vi "TLMB_Get_Latest_Build_From_Artifactory.vi"(7 "Repository":string="CIBuild_TLMB", 11 "Error In":errorcluster) -> (4 "Output Path":path, 8 "Build":string, 15 "Error Out 2":errorcluster)   [LabVIEW 2016, in "TLMB.lvlib"]
uses:
  Projects/TLMB.lvlib
  <vilib>/regexp/Match Regular Expression.xnode
  <vilib>/httpClient/LabVIEWHTTPClient.lvlib
  <vilib>/zip/NI_Unzip.lvlib
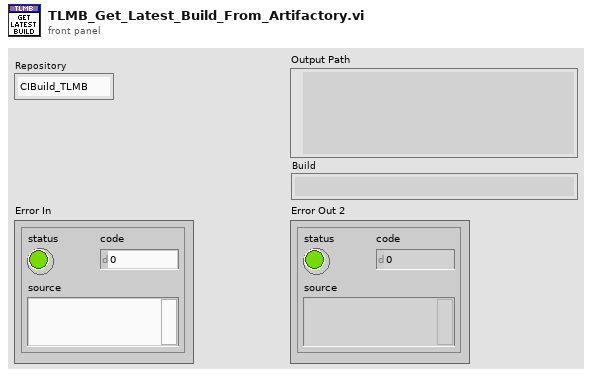
[diagram p1: front panel]
types:
  T1 = typedef "LabVIEWHTTPClient.lvlib/ClientHandle.ctl" = refnum<k1>
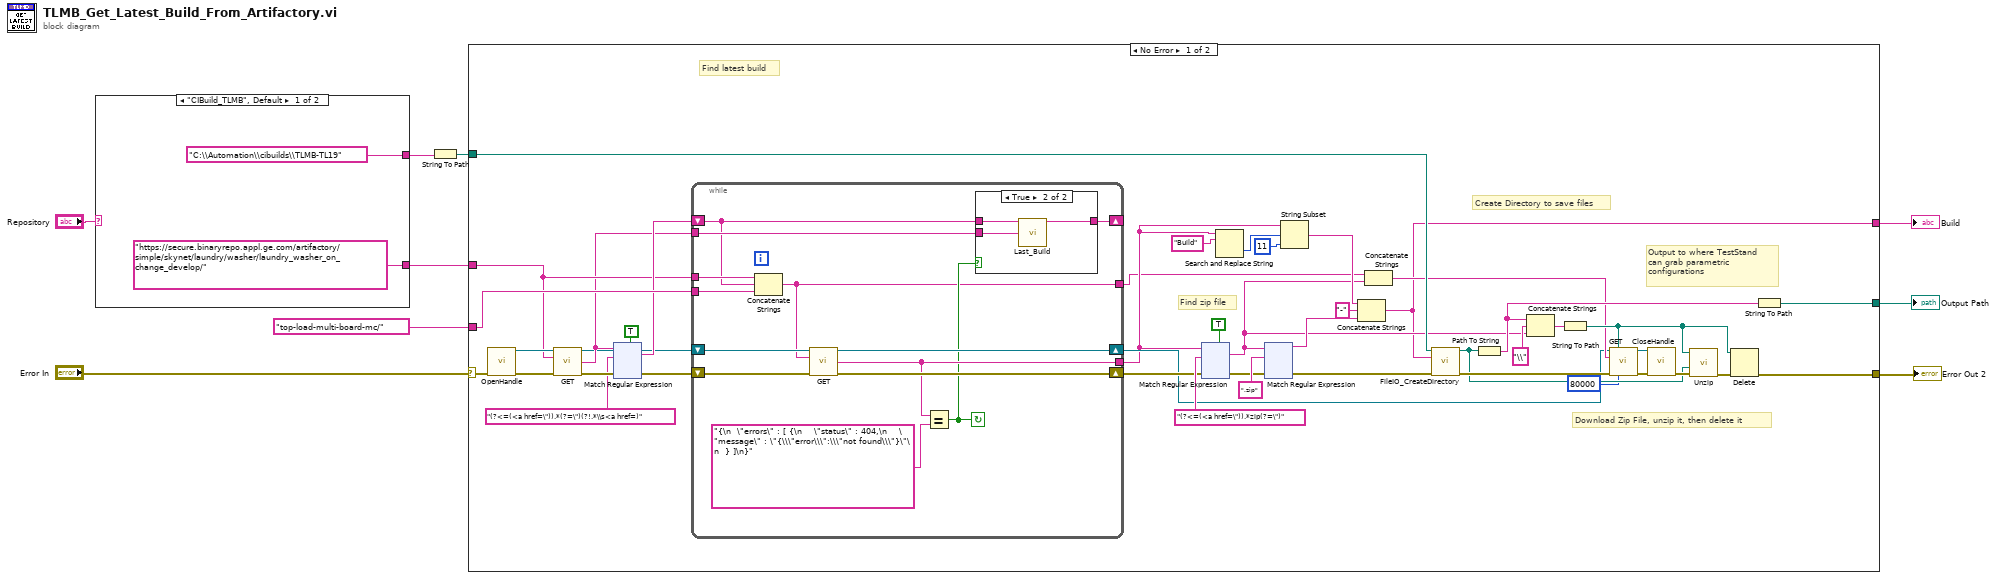
[diagram p0: block diagram]
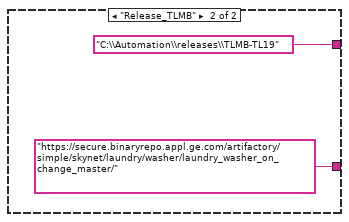
[diagram p2: hidden frame]
diagram:
  n1 = case shown="\"CIBuild_TLMB\", Default" "Repository" {
    tunnel: ["C:\\Automation\\cibuilds\\TLMB-TL19" "C:\\Automation\\releases\\TLMB-TL19"] -> w6
    tunnel: ["https://secure.binaryrepo.appl.ge.com/artifactory/simple/skynet/laundry/washer/laundry_washer_on_change_develop/" ("regular expression") "https://secure.binaryrepo.appl.ge.com/artifactory/simple/skynet/laundry/washer/laundry_washer_on_change_master/" ("regular expression")] -> w3
    frame "CIBuild_TLMB", Default {
    }
    frame "Release_TLMB" {
    }
  }
  n2 = String To Path(string=w6) -> (path=w5:path)
  n3 = case shown="No Error" "Error In" {
    selector: "Error In" -> [w55 w417]
    tunnel: [w40 w417] -> w7
    tunnel: [w35 _] -> w8
    tunnel: w5 -> [w36 _]
    tunnel: w3 -> [w21 _]
    tunnel: "top-load-multi-board-mc/" -> [w23 _]
    tunnel: [w24 _] -> w1
    frame No Error {
      # "Create Directory to save files"
      # "Output to where TestStand\ncan grab parametric\nconfigurations"
      # "Find zip file"
      # "Find latest build"
      # "Download Zip File, unzip it, then delete it"
      n4 = call <vilib>:"OpenHandle.vi"("error in (no error)"=w55) -> ("client handle out"=w56:T1, "error out"=w57:errorcluster)  [unwired: 13 in]
      n5 = call <vilib>:"GET.vi"("client handle"=w56, "url"=w21, "error in (no error)"=w57) -> ("client handle out"=w18:T1, "body"=w20:string, "error out"=w54:errorcluster)  [unwired: 9 in, 1 out]
      n6 = xnode "Match Regular Expression"("input string"=w20, "regular expression"="(?<=(<a href=\")).*(?=\")(?!.*\\s<a href=)", "error in"=w54, "multiline? (F)"=TRUE) -> ("whole match"=w22:string, "error out"=w19:errorcluster)  [unwired: 2 in, 3 out]
      n7 = while {
        shift-right: [w70] -> w17
        shift-left: w19 -> [w68]
        shift-right: [w69] -> w16
        shift-left: w18 -> [w67]
        tunnel: [w65] -> w15
        tunnel: w20 -> [w63]
        shift-right: [w62] -> _
        shift-left: w22 -> [w60]
        tunnel: w21 -> [w61]
        tunnel: [w59] -> w14
        tunnel: w23 -> [w58]
        stop <- w64 continue-if-true
        n8 = Concatenate Strings(w61, w60, w58) -> (w59:string)
        n9 = call <vilib>:"GET.vi"("client handle"=w67, "url"=w59, "error in (no error)"=w68) -> ("client handle out"=w69:T1, "body"=w65:string, "error out"=w70:errorcluster)  [unwired: 9 in, 1 out]
        n10 = Equal?(x=w65, y="{\n  \"errors\" : [ {\n    \"status\" : 404,\n    \"message\" : \"{\\\"error\\\":\\\"not found\\\"}\"\n  } ]\n}") -> (x = y?=w64:bool)
        n11 = case shown="True" w64 {
          tunnel: w63 -> [_ w74]
          tunnel: w60 -> [w71 w73]
          tunnel: [w71 w72] -> w62
          frame False {
          }
          frame True {
            n12 = call "Last_Build.vi"("Current Build"=w73, "Webpage Source"=w74) -> ("Next Build"=w72:string)  [unwired: 13 in]
          }
        }
      }
      n13 = xnode "Match Regular Expression"("input string"=w15, "regular expression"="(?<=(<a href=\")).*zip(?=\")", "error in"=w17, "multiline? (F)"=TRUE) -> ("whole match"=w26:string, "error out"=w44:errorcluster)  [unwired: 2 in, 3 out]
      n14 = Search and Replace String(input string=w15, search string="Build") -> (offset past replacement=w30:i32)  [unwired: 6 in, 3 out]
      n15 = xnode "Match Regular Expression"("input string"=w26, "regular expression"=".zip", "error in"=w44) -> ("before match"=w27:string, "error out"=w43:errorcluster)  [unwired: 3 in, 3 out]
      n16 = String Subset(string=w15, offset (0)=w30, length (rest)=11 ("length (rest)")) -> (substring=w28:string)
      n17 = Concatenate Strings(w28, "-" ("string"), w27) -> (w24:string)
      n18 = Concatenate Strings(w14, w26) -> (w25:string)
      n19 = call "FileIO_CreateDirectory.vi"("Base Path"=w36, "Directory Name"=w24, "Error In"=w43) -> ("File Path Control"=w39:path, "Error Out"=w46:errorcluster)  [unwired: 11 in]
      n20 = Path To String(path=w39) -> (string=w33:string)
      n21 = Concatenate Strings(w33, "\\" ("string"), w26) -> (w41:string)
      n22 = String To Path(string=w41) -> (path=w38:path)
      n23 = call <vilib>:"GET.vi"("client handle"=w16, "output file"=w38, "url"=w25, "error in (no error)"=w46, "timeout (10000)"=80000) -> ("client handle out"=w49:T1, "error out"=w48:errorcluster)  [unwired: 7 in, 2 out]
      n24 = call <vilib>:"CloseHandle.vi"("client handle"=w49, "error in (no error)"=w48) -> ("error out"=w47:errorcluster)  [unwired: 13 in]
      n25 = call <vilib>:"Unzip.vi"("error in (no error)"=w47, "Target directory (same as Zip file if empty)"=w39, "Zip file"=w38) -> ("error out"=w37:errorcluster)  [unwired: 6 in, 2 out]
      n26 = Delete(path (use dialog)=w38, error in=w37) -> (error out=w40:errorcluster)  [unwired: 3 in, 2 out]
      n27 = String To Path(string=w33) -> (path=w35:path)
    }
    frame Error {
    }
  }
  "Output Path" <- w8
  "Error Out 2" <- w7
  "Build" <- w1
